vi "Dash Tote Height.vi"   [LabVIEW 2014]
uses:
  <vilib>/Rock Robotics/Network Tables/SD Read Number.vi
  <vilib>/Rock Robotics/Network Tables/SD Read Boolean.vi
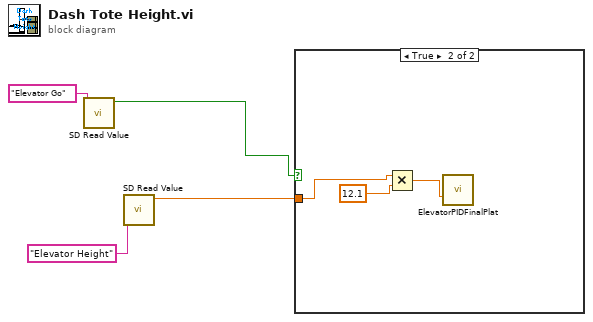
[diagram p0: block diagram]
diagram:
  n1 = call-poly <vilib>:"SD Read Value.vi"("Name"="Elevator Go") -> ("Boolean"=w2:bool)  [unwired: 8 in, 2 out]
  n2 = call-poly <vilib>:"SD Read Value.vi"("Name"="Elevator Height") -> ("Numeric"=w1:dbl)  [unwired: 8 in, 2 out]
  n3 = case shown="True" w2 {
    tunnel: w1 -> [_ w6]
    frame False {
    }
    frame True {
      n4 = Multiply(x=w6, y=12.1 ("Elevator Setpoint")) -> (x*y=w5:dbl)
      n5 = call "ElevatorPIDFinalPlat.vi"("Elevator Setpoint"=w5) -> ()  [unwired: 14 in, 1 out]
    }
  }
